vi "Inverse Filter, A-Weight Demo.vi"() -> ()   [LabVIEW 2015]
uses:
  Waveform VIs/Noise VIs/Noise Params.ctl
  Controls/Level XCtl/Level Data.ctl
  Controls/Level XCtl/Level Units.ctl
  Controls/Advanced Filter XCtl/Filter Data.ctl
  Filter VIs/Filter-Bandwidth Units.ctl
  Utility VIs/Math VIs/dB to Linear (1D).vi
  Utility VIs/Math VIs/FFT x(t) to dB,Degrees (1D).vi
  Utility VIs/Math VIs/dB to Linear (scalar).vi
  PXI DAQ VIs/DAQ Engine VIs/PXI Globals.vi
  Utility VIs/Math VIs/Linear to dB (scalar).vi
  Utility VIs/Math VIs/Linear to dB (array).vi
  Controls/Level XCtl/Level XCtl.xctl
  Controls/Advanced Filter XCtl/Advanced Filter XCtl.xctl
panel:
  in  "afile":path
  out "\"Theoretical\"":dbl
  out "Level (spectrum average)":dbl
  out "Max Level (forward filter)":dbl
  out "Noise through forward filter":cluster{"Frequency (Hz)":dbl[], "Mag":dbl[]}(graph)
  in  "Filter":T1={"Type"=enum."OFF", "CF (kHz)"=0.0, "BW (kHz)"=0.0, "Cascade"=FALSE, "Quadrature"=FALSE, "Scale Factor"=0.0, "Stages"=[], "Class"=enum."Elliptic", "Order"=0, "BWUnits"=enum."Linear"} {"Stages"."IIR Filter"."Forward Coefficients" format="%.4f"; "Stages"."IIR Filter"."Reverse Coefficients" format="%.4f"}
  in  "Level":T3={"Level"=0.0, "Units"=enum."dB SPL", "Max"=0.0, "Multiplier"=0.0, "Cal File"=path "", "Cal"={"Freq (Hz)"=[], "Mag (dB SPL)"=[], "Phase (deg)"=[]}}
  in  "Noise":T5={"InvFilt"=TRUE, "Noise"=[], "CurPt"=0, "Aweight"=FALSE, "Seed"=0, "afile"=path ""}
  in  "T (s)":dbl=0.1
  in  "Fs (Hz)":dbl=150000.0
  out "Noise spectrum":T6(graph)
  out "Calibration":cluster{"Frequency (Hz)":dbl[], "Mag":dbl[]}(graph)
  in  "Calibration file":path=path "D:/Data/XYZ DATA/XYZ999/LeftSecondary.calib"
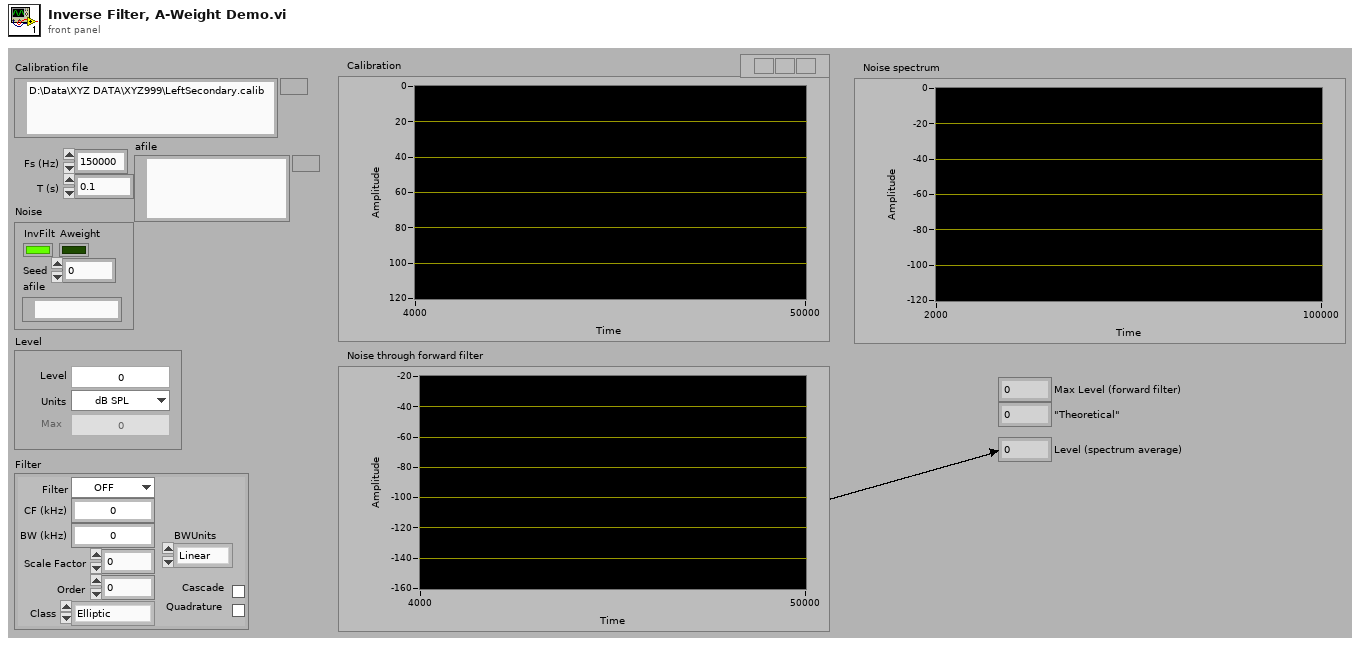
[diagram p1: front panel]
types:
  T1 = typedef "Advanced Filter XCtl.xctl/Filter Data.ctl" = cluster{"Type":enum16{"Lowpass", "Highpass", "Bandpass", "Bandstop", "OFF"}, "CF (kHz)":dbl, "BW (kHz)":dbl, "Cascade":bool, "Quadrature":bool, "Scale Factor":dbl, "Stages":cluster{"IIR Filter":cluster{"filter structure":enum32{"IIR 2nd Order", "IIR 4th Order"}, "Reverse Coefficients":dbl[], "Forward Coefficients":dbl[]}, "State":dbl[]}[], "Class":enum16{"Elliptic", "Butterworth"}, "Order":i32, "BWUnits":T2}
  T2 = typedef "Filter-Bandwidth Units.ctl" = enum16{"Linear", "Octaves", "Min-Max"}
  T3 = typedef "Level XCtl.xctl/Level Data.ctl" = cluster{"Level":dbl, "Units":T4, "Max":dbl, "Multiplier":dbl, "Cal File":path, "Cal":cluster{"Freq (Hz)":dbl[], "Mag (dB SPL)":dbl[], "Phase (deg)":dbl[]}}
  T4 = typedef "Level Units.ctl" = enum16{"dB atten", "dB SPL", "dB re 1 Vrms", "dB V/Hz½", "mW", "dB HL", "Volts", "dB mW"}
  T5 = typedef "Noise Params.ctl" = cluster{"InvFilt":bool, "Noise":dbl[], "CurPt":i32, "Aweight":bool, "Seed":i32, "afile":path}
  T6 = cluster{"Freq (Hz)":dbl[], "+Freq. Mag of FFT (dB rms)":dbl[]}
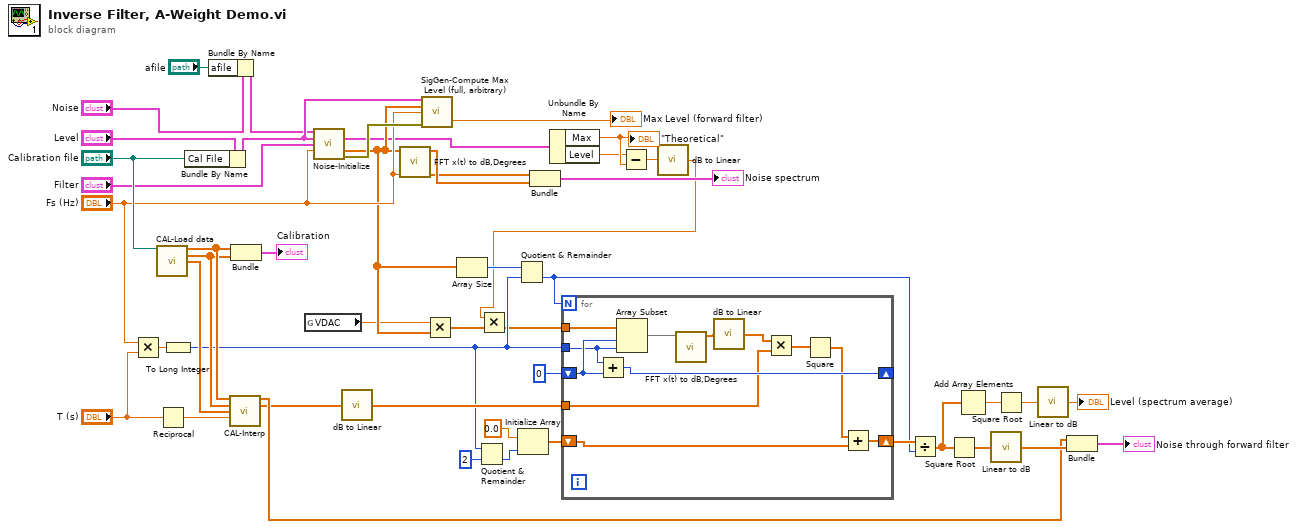
[diagram p0: block diagram]
diagram:
  n1 = Multiply(x="Fs (Hz)", y="T (s)") -> (x*y=w38:dbl)
  n2 = call "CAL-Load data.vi"("user path"="Calibration file") -> ("Frequency (Hz)"=w48:dbl[], "Mag"=w47:dbl[], "Phase"=w46:dbl[])  [unwired: 7 in, 5 out]
  n3 = Reciprocal(x="T (s)") -> (1/x=w45:dbl)
  n4 = To Long Integer(number=w38) -> (32bit integer=w27:i32)
  n5 = Bundle By Name(cluster="Level", "Cal File"="Calibration file") -> (w16:T3)
  n6 = Bundle By Name(cluster="Noise", "afile"="afile") -> (w2:T5)
  n7 = call "CAL-Interp.vi"("Frequency (Hz)"=w48, "Magnitude (dB)"=w47, "Phase (degrees)"=w46, "df (Hz)"=w45) -> ("Interp Freq (Hz)"=w30:dbl[], "Interp Magnitude (dB)"=w29:dbl[])  [unwired: 8 in, 2 out]
  n8 = Bundle("Frequency (Hz)"=w48, "Mag"=w47) -> (→"Calibration":cluster{"Frequency (Hz)":dbl[], "Mag":dbl[]})  [unwired: 1 in]
  n9 = global read "PXI Globals.vi" "VDAC"() -> (w8:dbl)
  n10 = call "Noise-Initialize.vi"("Noise"=w2, "Level"=w16, "Filter"="Filter", "Sampling rate (Hz)"="Fs (Hz)") -> ("Level Out"=w9:T3, "Noise"=w17:dbl[], "error out"=w19:errorcluster)  [unwired: 7 in, 2 out]
  n11 = call-poly "dB to Linear.vi"("dB"=w29) -> ("linear"=w28:dbl[])
  n12 = call-poly "FFT x(t) to dB,Degrees.vi"("Fs (Hz)"="Fs (Hz)", "X"=w17) -> ("Freq (Hz)"=w40:dbl[], "+Freq. Mag of FFT (dB rms)"=w41:dbl[])  [unwired: 7 in, 1 out]
  n13 = call "SigGen-Compute Max Level (full, arbitrary).vi"("Level"=w16, "Y"=w17, "Sampling Rate (Hz)"="Fs (Hz)", "error in (no error)"=w19) -> ("Max Level"=→"Max Level (forward filter)":dbl)  [unwired: 9 in, 2 out]
  n14 = Multiply(x=w8, y=w17) -> (x*y=w10:dbl[])
  n15 = Array Size(array=w17) -> (size(s)=w37:i32)
  n16 = Quotient & Remainder(x=w27, y=2) -> (floor(x/y)=w36:i32)  [unwired: 1 out]
  n17 = Quotient & Remainder(x=w37, y=w27) -> (floor(x/y)=w25:i32)  [unwired: 1 out]
  n18 = Initialize Array(0.0, w36) -> (w33:dbl[])
  n19 = Bundle("Freq (Hz)"=w40, "+Freq. Mag of FFT (dB rms)"=w41) -> (→"Noise spectrum":T6)  [unwired: 1 in]
  n20 = Unbundle By Name(w9) -> ("Max"=w7:dbl, "Level"=w6:dbl)
  "\"Theoretical\"" <- w7
  n21 = Subtract(x=w6, y=w7) -> (x-y=w4:dbl)
  n22 = call-poly "dB to Linear.vi"("dB"=w4) -> ("linear"=w3:dbl)
  n23 = Multiply(x=w3, y=w10) -> (x*y=w5:dbl[])
  n24 = for {
    N: w25 -> [_]
    tunnel: w5 -> [w60]
    tunnel: w27 -> [w58]
    shift-right: [w57] -> _
    shift-left: 0 -> [w59]
    tunnel: w28 -> [w56]
    shift-right: [w52] -> w32
    shift-left: w33 -> [w53]
    n25 = Add(x=w58, y=w59) -> (x+y=w57:i32)
    n26 = Array Subset(array=w60, index=w59, length=w58) -> (w49:dbl[])
    n27 = call-poly "FFT x(t) to dB,Degrees.vi"("X"=w49) -> ("+Freq. Mag of FFT (dB rms)"=w51:dbl[])  [unwired: 8 in, 2 out]
    n28 = call-poly "dB to Linear.vi"("dB"=w51) -> ("linear"=w50:dbl[])
    n29 = Multiply(x=w50, y=w56) -> (x*y=w55:dbl[])
    n30 = Square(x=w55) -> (x^2=w54:dbl[])
    n31 = Add(x=w54, y=w53) -> (x+y=w52:dbl[])
  }
  n32 = Divide(x=w32, y=w25) -> (x/y=w14:dbl[])
  n33 = Square Root(x=w14) -> (sqrt(x)=w21:dbl[])
  n34 = Add Array Elements(numeric array=w14) -> (sum=w12:dbl)
  n35 = call-poly "Linear to dB.vi"("linear"=w21) -> ("dB"=w31:dbl[])
  n36 = Square Root(x=w12) -> (sqrt(x)=w13:dbl)
  n37 = call-poly "Linear to dB.vi"("Linear"=w13) -> ("dB"=→"Level (spectrum average)":dbl)
  n38 = Bundle("Interp Freq (Hz)"=w30, "dB"=w31) -> (→"Noise through forward filter":cluster{"Interp Freq (Hz)":dbl[], "dB":dbl[]})  [unwired: 1 in]
